vi "UnbundleDatesToNumber.vi"(5 "Cluster":T1 {"Start" format="%<%.3X>T"}) -> (0 "End":dbl, 1 "Start":dbl, 2 "String":string)   [LabVIEW 2017]
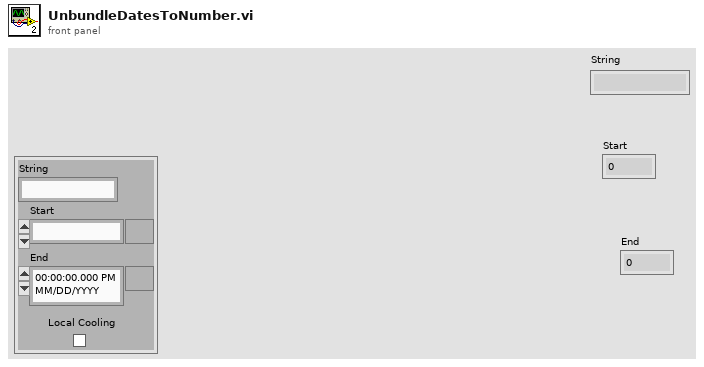
[diagram p1: front panel]
types:
  T1 = cluster{"String":string, "Start":timestamp, "End":timestamp, "Local Cooling":bool}
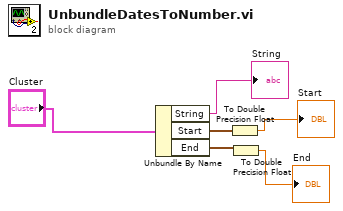
[diagram p0: block diagram]
diagram:
  n1 = Unbundle By Name("Cluster") -> ("String"=→"String":string, "Start"=w5:timestamp, "End"=w4:timestamp)
  n2 = To Double Precision Float(number=w5) -> (double precision float=→"Start":dbl)
  n3 = To Double Precision Float(number=w4) -> (double precision float=→"End":dbl)
